vi "Get_fileName.vi"(8 "error in (no error)":errorcluster caption="错误输入（无错误）", 11 "VISA资源名称":refnum<visa-resource-name>) -> (0 "error out":errorcluster caption="错误输出", 1 "读取缓冲区":string, 3 "VISA资源名称输出":refnum<visa-resource-name>)   [LabVIEW 2018]
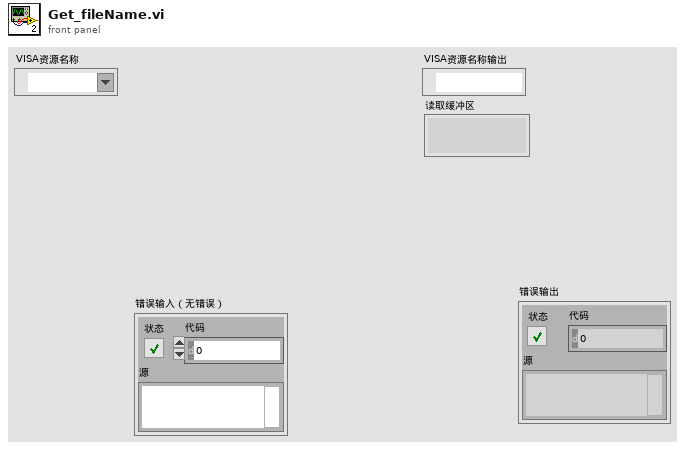
[diagram p1: front panel]
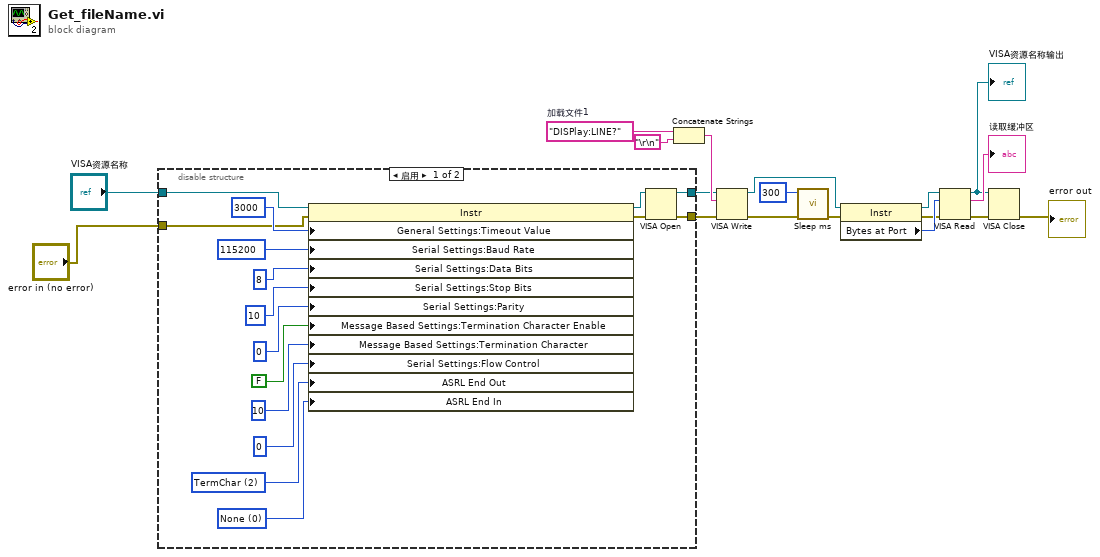
[diagram p0: block diagram]
diagram:
  w18 = "DISPlay:LINE?"  # 加载文件1
  n1 = disable-structure shown="启用" {
    disable-tunnel: [w34 w35] -> w6
    disable-tunnel: [w33 _] -> w5
    disable-tunnel: "VISA资源名称" -> [w30 w35]
    disable-tunnel: "error in (no error)" -> [w19 _]
    frame Enabled {
      w24 = u16 0 items=["None", "Last Bit", "TermChar"] ("Serial Settings:End Mode for Reads")
      w26 = u16 2 items=["None", "Last Bit", "TermChar", "Break"] ("Serial Settings:End Mode for Writes")
      n2 = property class="Instr"(reference=w30, error in=w19, "General Settings:Timeout Value"=u32 3000, "Serial Settings:Baud Rate"=u32 115200, "Serial Settings:Data Bits"=u16 8, "Serial Settings:Stop Bits"=u16 10, "Serial Settings:Parity"=u16 0, "Message Based Settings:Termination Character Enable"=FALSE ("TermChar En"), "Message Based Settings:Termination Character"=u8 10, "Serial Settings:Flow Control"=u16 0, "ASRL End Out"=w26, "ASRL End In"=w24) -> (reference out=w31:refnum<visa-resource-name>, error out=w32:errorcluster)
      n3 = VISA Open ("VISA打开")(error in (no error)=w32, VISA resource name=w31) -> (VISA resource name=w34:refnum<visa-resource-name>, error out=w33:errorcluster)  [unwired: 3 in]
    }
    frame Disabled {
    }
  }
  n4 = Concatenate Strings(w18, "\r\n") -> (w16:string)
  n5 = VISA Write(VISA resource name=w6, write buffer=w16, error in (no error)=w5) -> (VISA resource name out=w15:refnum<visa-resource-name>, error out=w12:errorcluster)  [unwired: 1 out]
  n6 = call "Sleep ms.vi"("error in (no error)"=w12, "等待时间（毫秒）"=u32 300) -> ("error out"=w4:errorcluster)  [unwired: 9 in]
  n7 = property class="Instr"(reference=w15, error in=w4) -> (reference out=w13:refnum<visa-resource-name>, error out=w11:errorcluster, "Bytes at Port"=w14:u32)
  n8 = VISA Read(VISA resource name=w13, byte count=w14, error in (no error)=w11) -> (VISA resource name out=w8:refnum<visa-resource-name>, read buffer=→"读取缓冲区":string, error out=w9:errorcluster)  [unwired: 1 out]
  "VISA资源名称输出" <- w8
  n9 = VISA Close(VISA resource name=w8, error in (no error)=w9) -> (error out=→"error out":errorcluster)
